vi "tui_LuaVIEW Function Manager.vi"() -> ()   [LabVIEW 2012]
doc: "A manager for Lua-callable functions. It supports LuaVIEW function VIs as well as functions with a doc string contained in function library scripts. The documentation of individual functions can be shown. Overview documentation of the listed functions can be exported to HTML. When running under the LabVIEW development environment, function VIs and their documentation can be opened and edited."
uses:
  served/LuaVIEW Loaded Function Infos_srv.ctl
  served/LuaVIEW Get Function Documentation_srv.ctl
  served/LuaVIEW Cleanup Registry_srv.ctl
  typedefs/t_LuaVIEW Function Manager States.ctl
  library/typedefs/t_Library Session Methods.ctl
  clientsrv/typedefs/t_ClientSrv Access Levels.ctl
  typedefs/clusters/LuaVIEW Function Info.ctl
panel:
  out "cleanup registry":T1
  in  "cleanup":bool
  out "llb path cache":path
  out "new selection":T2(ring)
  out "html paths":path[](array[path])
  out "library path cache":path
  out "base path cache":path
  out "source selection":T2(ring)
  in  "function source":u16(ring) items=["select", "loaded on server", "base directory", "VI library", "function library"]
  out "source":string
  in  "function filter":string
  in  "refresh":bool
  out "get func doc":T3
  in  "edit":bool
  in  "open":bool
  in  "export":bool
  in  "show":bool
  out "loaded func infos":T4
  in  "function list":i32(listbox)
  in  "exit":bool
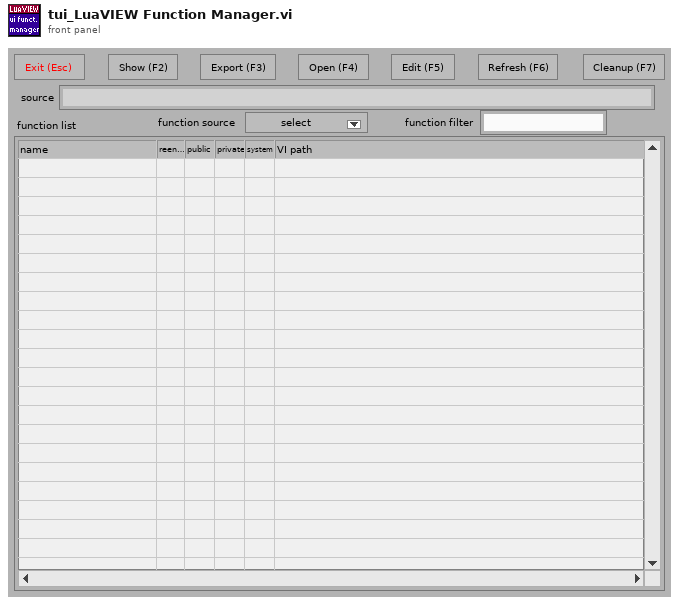
[diagram p1: front panel]
types:
  T1 = typedef "LuaVIEW Cleanup Registry_srv.ctl" = refnum<vi>
  T2 = enum16{"loaded on server", "base directory", "VI library", "function library"}
  T3 = typedef "LuaVIEW Get Function Documentation_srv.ctl" = refnum<vi>
  T4 = typedef "LuaVIEW Loaded Function Infos_srv.ctl" = refnum<vi>
  T5 = typedef "t_LuaVIEW Function Manager States.ctl" = enum16{"empty queue", "update source", "set source", "refresh source", "cleanup registry", "update list", "update ablement", "show", "export", "open", "edit", "fetch loaded", "query base", "query llb", "recurse base", "query library", "parse library", "match sizes", "initialize", "init refs", "init disable", "init persist", "init source", "cleanup", "stop"}
  T6 = typedef "t_Library Session Methods.ctl" = enum16{"run", "get arg", "set arg", "delist", "cleanup?", "start session", "stop session", "list empty?"}
  T7 = typedef "t_ClientSrv Access Levels.ctl" = enum16{"observer", "operator", "local"}
  T8 = typedef "LuaVIEW Function Info.ctl" = cluster{"path":path, "reentrant":bool, "public":bool, "private":i32, "system":bool, "other path":bool, "name":string, "docstring":string, "synopsis":string}
  T9 = typedef "eventvkey.ctl" = enum16{"ASCII", "Enter", "Return", "Shift", "Ctrl", "Alt", "Cmd", "Opt", "Caps", "NumLock", "Clear", "Break", "Up", "Down", "Left", "Right", "Insert", "Delete", "Home", "End", "PageUp", "PageDown", "Escape", "Help", "Pause", "ScrollLock", "F1", "F2", "F3", "F4", "F5", "F6", "F7", "F8", "F9", "F10", "F11", "F12", "F13", "F14", "F15", "F16", "F17", "F18", "F19", "F20", "F21", "F22", "F23", "F24", "Play", "VolumeUp", "VolumeDown", "Mute", "Two Byte Char"}
  T10 = enum32{"invalid app kind", "Development System", "Run Time System", "Student Edition", "Embedded LabVIEW", "Evaluation", "Custom"}
  T11 = enum32{"existing file", "new file", "new or existing file", "existing dir", "new dir", "new or existing dir", "existing file (use LLBs)", "new file (use LLBs)", "new or existing file (use LLBs)", "new or existing file or directory (use LLBs)"}
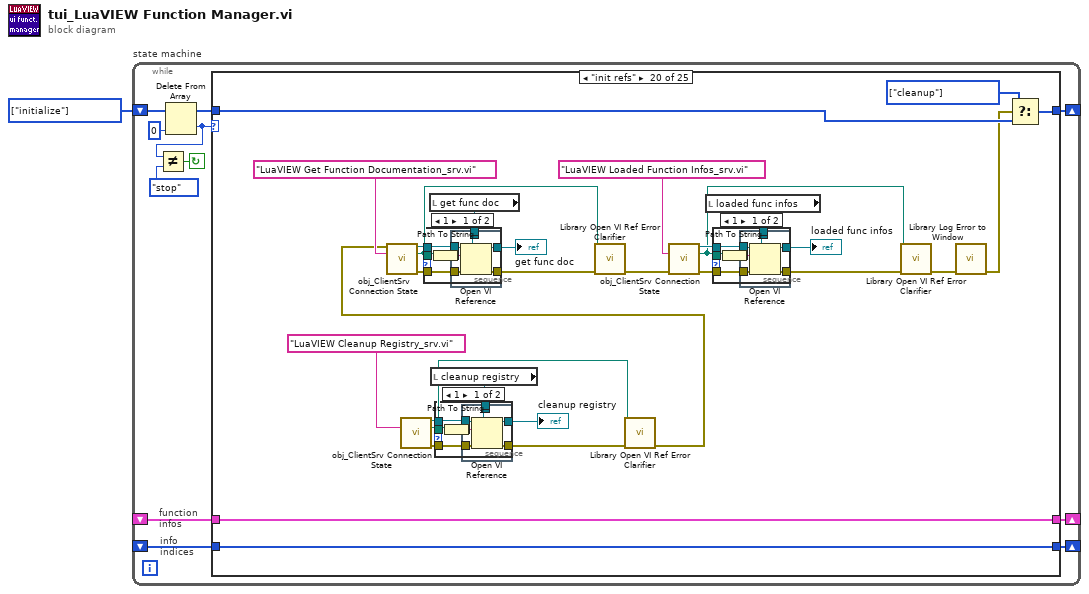
[diagram p0: block diagram]
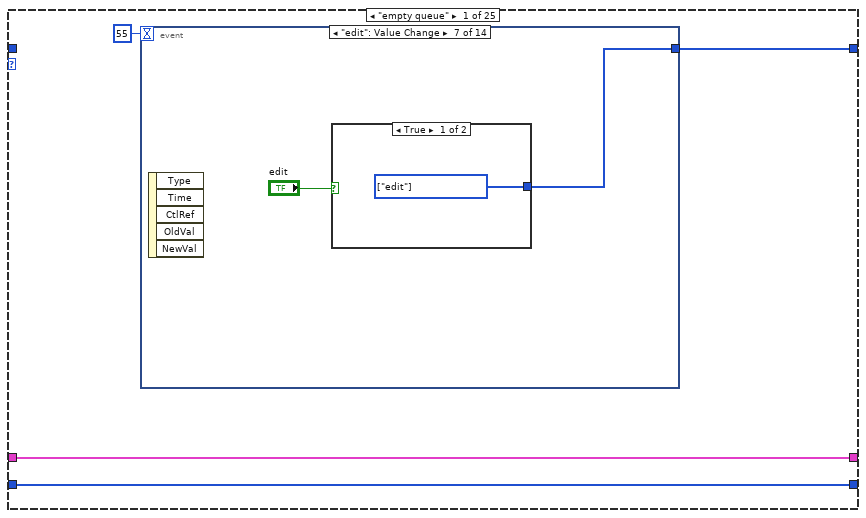
[diagram p2: hidden frame]
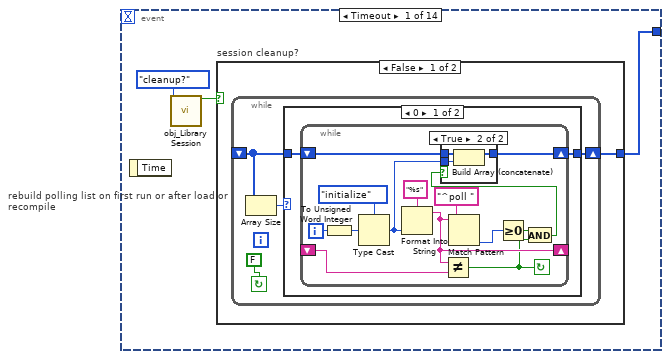
[diagram p3: hidden frame]
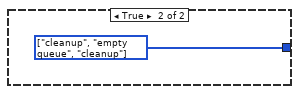
[diagram p6: hidden frame]
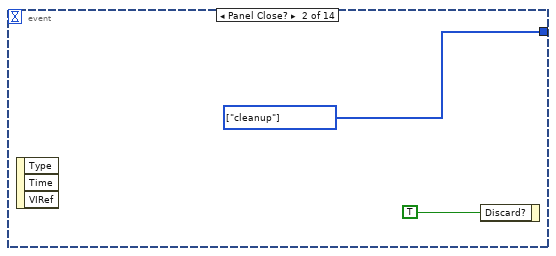
[diagram p7: hidden frame]
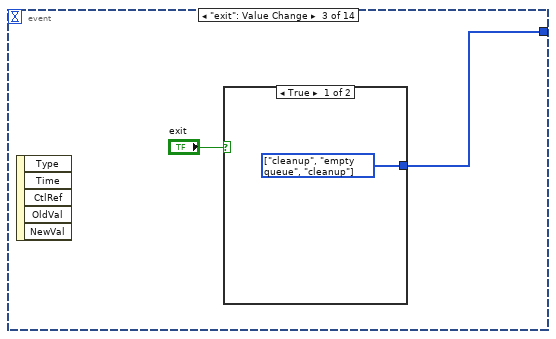
[diagram p8: hidden frame]
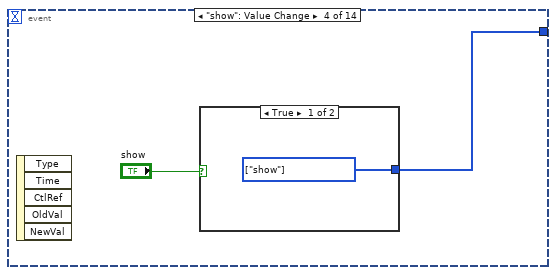
[diagram p10: hidden frame]
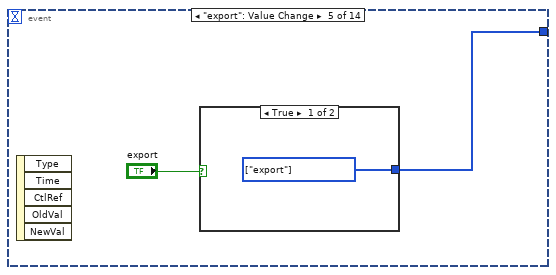
[diagram p12: hidden frame]
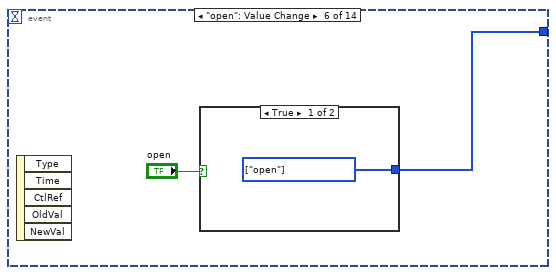
[diagram p14: hidden frame]
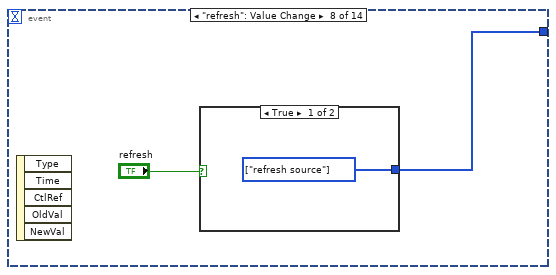
[diagram p17: hidden frame]
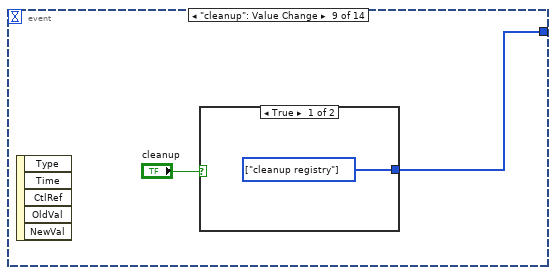
[diagram p19: hidden frame]
diagram:
  w1 = T5[] [enum."initialize"] items=["empty queue", "update source", "set source", "refresh source", "cleanup registry", "update list", "update ablement", "show", "export", "open", "edit", "fetch loaded", "query base", "query llb", "recurse base", "query library", "parse library", "match sizes", "initialize", "init refs", "init disable", "init persist", "init source", "cleanup", "stop"] ("Array Constant")
  n1 = while "state machine" {
    shift-left: w1 -> [w9]
    shift-right: [w12] -> _
    shift-right: [w4] -> _
    shift-left: _ -> [w5]
    shift-right: [w2] -> _
    shift-left: _ -> [w3]
    stop <- w11 continue-if-true
    # "info\nindices"
    # "function\ninfos"
    n2 = Delete From Array(array=w9, index=0) -> (deleted portion=w6:T5, array with subset deleted=w8:T5[])  [unwired: 1 in]
    n3 = Not Equal?(x=w6, y=t_LuaVIEW_Function_Manager_States."stop" ("states")) -> (x != y?=w11:bool)
    n4 = case "Case" shown="\"init refs\"" w6 {
      tunnel: [w16 w98 w105 w109 w124 w141 w214 w231 w268 w380 w394 w405 w430 w443 w453 w477 w488 w502 w507 w562 w629 w631 w651 w660 w663] -> w12
      tunnel: w8 -> [_ _ w105 w108 _ w146 w214 w231 w268 w380 w394 w406 w432 w445 w452 w479 w487 w502 _ w560 w629 w634 w650 _ w663]
      tunnel: w5 -> [w15 w99 w106 w113 w126 w145 w210 w227 w263 w375 w389 _ w431 w444 _ w478 _ w504 w506 w559 w627 w633 w649 w656 w662]
      tunnel: [w15 w99 w106 w113 w126 w145 w210 w227 w263 w375 w389 w407 w431 w444 w454 w478 w489 w504 w506 w559 w627 w633 w647 w656 w662] -> w4
      tunnel: w3 -> [w14 w97 w107 w111 w125 _ w213 w229 w262 w374 w390 w403 w428 w441 w449 w475 w484 w503 w505 w558 w626 w632 w644 w655 w661]
      tunnel: [w14 w97 w107 w111 w125 w142 w213 w229 w262 w374 w390 w403 w428 w441 w449 w475 w484 w503 w505 w558 w626 w632 w643 w655 w661] -> w2
      frame "empty queue" {
        n5 = event shown="[6] \"edit\": Value Change" {
          selector: _ -> [_ _ _ _ _ _ _ _ _ _ _ _ _ _]
          dyn-events: _ -> [_ _ _ _ _ _ _ _ _ _ _ _ _ _]
          timeout: 55 -> [_ _ _ _ _ _ _ _ _ _ _ _ _ _]
          tunnel: [w19 w48 w50 w53 w56 w59 w62 w65 w68 w72 w83 w86 w91 _] -> w16
          event Timeout {
            n6 = event-data() -> ()  [unwired: 1 in, 1 out]
            n7 = call "obj_Library Session.vi"("method"=t_Library_Session_Methods."cleanup?") -> ("cleanup/empty?"=w18:bool)  [unwired: 11 in, 3 out]
            n8 = case "session cleanup?" shown="False" w18 {
              tunnel: [w20 w46] -> w19
              frame False {
                n9 = while "rebuild polling list on first run or after load or recompile" {
                  shift-left: _ -> [w23]
                  shift-right: [w22] -> w20
                  stop <- FALSE continue-if-true
                  n10 = Array Size(array=w23) -> (size(s)=w24:i32)
                  n11 = case shown="0" w24 {
                    tunnel: [w25 w45] -> w22
                    tunnel: w23 -> [w26 w45]
                    frame 0 {
                      n12 = while {
                        shift-left: w26 -> [w35]
                        shift-right: [w33] -> w25
                        shift-left: _ -> [w37]
                        shift-right: [w32] -> _
                        i -> [w40]
                        stop <- w28 continue-if-true
                        n13 = To Unsigned Word Integer(number=w40) -> (unsigned 16bit integer=w38:u16)
                        n14 = Type Cast(type=t_LuaVIEW_Function_Manager_States."initialize" ("states"), x=w38) -> (*(type *) &x=w34:T5)
                        n15 = Format Into String(format string="%s" ("Format String"), w34) -> (resulting string=w32:string)  [unwired: 2 in, 1 out]
                        n16 = Not Equal?(x=w32, y=w37) -> (x != y?=w28:bool)
                        n17 = Match Pattern(string=w32, regular expression="^poll ") -> (offset past match=w30:i32)  [unwired: 1 in, 3 out]
                        n18 = Greater Or Equal To 0?(x=w30) -> (x >= 0?=w29:bool)
                        n19 = And(x=w29, y=w28) -> (x .and. y?=w27:bool)
                        n20 = case shown="True" w27 {
                          tunnel: w35 -> [w41 w44]
                          tunnel: w34 -> [_ w43]
                          tunnel: [w41 w42] -> w33
                          frame False {
                          }
                          frame True {
                            n21 = Build Array (concatenate)(w44, w43) -> (w42:T5[])
                          }
                        }
                      }
                    }
                    frame Default {
                    }
                  }
                }
              }
              frame True {
                w46 = T5[] [enum."cleanup", enum."empty queue", enum."cleanup"] items=["empty queue", "update source", "set source", "refresh source", "cleanup registry", "update list", "update ablement", "show", "export", "open", "edit", "fetch loaded", "query base", "query llb", "recurse base", "query library", "parse library", "match sizes", "initialize", "init refs", "init disable", "init persist", "init source", "cleanup", "stop"] ("Array Constant")
              }
            }
          }
          event Panel Close? {
            w48 = T5[] [enum."cleanup"] items=["empty queue", "update source", "set source", "refresh source", "cleanup registry", "update list", "update ablement", "show", "export", "open", "edit", "fetch loaded", "query base", "query llb", "recurse base", "query library", "parse library", "match sizes", "initialize", "init refs", "init disable", "init persist", "init source", "cleanup", "stop"] ("Array Constant")
            n22 = event-data() -> ()  [unwired: 1 in, 3 out]
            n23 = event-data("Discard?"=TRUE) -> ()  [unwired: 1 in, 1 out]
          }
          event "exit": Value Change {
            n24 = event-data() -> ()  [unwired: 1 in, 5 out]
            n25 = case shown="True" "exit" {
              tunnel: [w51 _] -> w50
              frame True {
                w51 = T5[] [enum."cleanup", enum."empty queue", enum."cleanup"] items=["empty queue", "update source", "set source", "refresh source", "cleanup registry", "update list", "update ablement", "show", "export", "open", "edit", "fetch loaded", "query base", "query llb", "recurse base", "query library", "parse library", "match sizes", "initialize", "init refs", "init disable", "init persist", "init source", "cleanup", "stop"] ("Array Constant")
              }
              frame False {
              }
            }
          }
          event "show": Value Change {
            n26 = event-data() -> ()  [unwired: 1 in, 5 out]
            n27 = case shown="True" "show" {
              tunnel: [w54 _] -> w53
              frame True {
                w54 = T5[] [enum."show"] items=["empty queue", "update source", "set source", "refresh source", "cleanup registry", "update list", "update ablement", "show", "export", "open", "edit", "fetch loaded", "query base", "query llb", "recurse base", "query library", "parse library", "match sizes", "initialize", "init refs", "init disable", "init persist", "init source", "cleanup", "stop"] ("Array Constant")
              }
              frame False {
              }
            }
          }
          event "export": Value Change {
            n28 = event-data() -> ()  [unwired: 1 in, 5 out]
            n29 = case shown="True" "export" {
              tunnel: [w57 _] -> w56
              frame True {
                w57 = T5[] [enum."export"] items=["empty queue", "update source", "set source", "refresh source", "cleanup registry", "update list", "update ablement", "show", "export", "open", "edit", "fetch loaded", "query base", "query llb", "recurse base", "query library", "parse library", "match sizes", "initialize", "init refs", "init disable", "init persist", "init source", "cleanup", "stop"] ("Array Constant")
              }
              frame False {
              }
            }
          }
          event "open": Value Change {
            n30 = event-data() -> ()  [unwired: 1 in, 5 out]
            n31 = case shown="True" "open" {
              tunnel: [w60 _] -> w59
              frame True {
                w60 = T5[] [enum."open"] items=["empty queue", "update source", "set source", "refresh source", "cleanup registry", "update list", "update ablement", "show", "export", "open", "edit", "fetch loaded", "query base", "query llb", "recurse base", "query library", "parse library", "match sizes", "initialize", "init refs", "init disable", "init persist", "init source", "cleanup", "stop"] ("Array Constant")
              }
              frame False {
              }
            }
          }
          event "edit": Value Change {
            n32 = event-data() -> ()  [unwired: 1 in, 5 out]
            n33 = case shown="True" "edit" {
              tunnel: [w63 _] -> w62
              frame True {
                w63 = T5[] [enum."edit"] items=["empty queue", "update source", "set source", "refresh source", "cleanup registry", "update list", "update ablement", "show", "export", "open", "edit", "fetch loaded", "query base", "query llb", "recurse base", "query library", "parse library", "match sizes", "initialize", "init refs", "init disable", "init persist", "init source", "cleanup", "stop"] ("Array Constant")
              }
              frame False {
              }
            }
          }
          event "refresh": Value Change {
            n34 = event-data() -> ()  [unwired: 1 in, 5 out]
            n35 = case shown="True" "refresh" {
              tunnel: [w66 _] -> w65
              frame True {
                w66 = T5[] [enum."refresh source"] items=["empty queue", "update source", "set source", "refresh source", "cleanup registry", "update list", "update ablement", "show", "export", "open", "edit", "fetch loaded", "query base", "query llb", "recurse base", "query library", "parse library", "match sizes", "initialize", "init refs", "init disable", "init persist", "init source", "cleanup", "stop"] ("Array Constant")
              }
              frame False {
              }
            }
          }
          event "cleanup": Value Change {
            n36 = event-data() -> ()  [unwired: 1 in, 5 out]
            n37 = case shown="True" "cleanup" {
              tunnel: [w69 _] -> w68
              frame True {
                w69 = T5[] [enum."cleanup registry"] items=["empty queue", "update source", "set source", "refresh source", "cleanup registry", "update list", "update ablement", "show", "export", "open", "edit", "fetch loaded", "query base", "query llb", "recurse base", "query library", "parse library", "match sizes", "initialize", "init refs", "init disable", "init persist", "init source", "cleanup", "stop"] ("Array Constant")
              }
              frame False {
              }
            }
          }
          event Key Down? {
            n38 = event-data() -> ("VKey"=w70:T9, "FocusObj"=w71:refnum<vi>)  [unwired: 1 in, 6 out]
            n39 = call <vilib>:"compatReturnToEnter.vi"("VKey"=w70) -> ("VKey"=w74:T9)
            n40 = case shown="\"Up\", \"Down\"" w74 {
              tunnel: [_ TRUE TRUE _] -> w73
              tunnel: [_ _ w81 _] -> w72
              tunnel: w71 -> [w76 _ _ _]
              frame "Up", "Down" {
                n41 = Type Cast(type=u32 0, x=w76) -> (*(type *) &x=w77:u32)
                n42 = Equal To 0?(x=w77) -> (x = 0?=w75:bool)
                n43 = case shown="True" w75 {
                  frame False {
                  }
                  frame True {
                    n44 = property on="function list" class="MCListbox (strict)"("Key Focus"=TRUE) -> ()  [unwired: 2 in, 2 out]
                  }
                }
              }
              frame "F1" {
                n45 = call "Library Show Help.vi"() -> ()  [unwired: 1 in]
              }
              frame "Enter" {
                w81 = T5[] [enum."show"] items=["empty queue", "update source", "set source", "refresh source", "cleanup registry", "update list", "update ablement", "show", "export", "open", "edit", "fetch loaded", "query base", "query llb", "recurse base", "query library", "parse library", "match sizes", "initialize", "init refs", "init disable", "init persist", "init source", "cleanup", "stop"] ("Array Constant")
              }
              frame Default {
              }
            }
            n46 = event-data("Discard?"=w73) -> ()  [unwired: 5 in, 1 out]
          }
          event "function filter": Value Change {
            w83 = T5[] [enum."update list"] items=["empty queue", "update source", "set source", "refresh source", "cleanup registry", "update list", "update ablement", "show", "export", "open", "edit", "fetch loaded", "query base", "query llb", "recurse base", "query library", "parse library", "match sizes", "initialize", "init refs", "init disable", "init persist", "init source", "cleanup", "stop"] ("Array Constant")
            n47 = event-data() -> ()  [unwired: 1 in, 5 out]
          }
          event "function source": Value Change {
            n48 = event-data() -> ()  [unwired: 1 in, 6 out]
            n49 = Greater Than 0?(x="function source") -> (x > 0?=w85:bool)
            n50 = case shown="True" w85 {
              tunnel: [_ w89] -> w86
              tunnel: "function source" -> [_ w88]
              frame False {
              }
              frame True {
                w89 = T5[] [enum."update source"] items=["empty queue", "update source", "set source", "refresh source", "cleanup registry", "update list", "update ablement", "show", "export", "open", "edit", "fetch loaded", "query base", "query llb", "recurse base", "query library", "parse library", "match sizes", "initialize", "init refs", "init disable", "init persist", "init source", "cleanup", "stop"] ("Array Constant")
                n51 = Decrement(x=w88) -> (x-1=→"new selection":u16)
                n52 = stacked-sequence {
                  tunnel: w88 -> [_]
                  frame #0 {
                    w90 = u16 0 items=["select", "loaded on server", "base directory", "function library"] ("function source")
                    n53 = local write "function source"(w90) -> ()
                  }
                }
              }
            }
          }
          event Panel Resize {
            w91 = T5[] [enum."match sizes"] items=["empty queue", "update source", "set source", "refresh source", "cleanup registry", "update list", "update ablement", "show", "export", "open", "edit", "fetch loaded", "query base", "query llb", "recurse base", "query library", "parse library", "match sizes", "initialize", "init refs", "init disable", "init persist", "init source", "cleanup", "stop"] ("Array Constant")
            n54 = event-data() -> ()  [unwired: 1 in, 8 out]
          }
          event event type 5.0.x8000000b {
            n55 = event-data() -> ("VKey"=w92:T9)  [unwired: 1 in, 9 out]
            n56 = call <vilib>:"compatReturnToEnter.vi"("VKey"=w92) -> ("VKey"=w94:T9)
            n57 = case shown="\"F1\"" w94 {
              tunnel: [_ TRUE] -> w93
              frame Default {
              }
              frame "F1" {
              }
            }
            n58 = event-data("Discard?"=w93) -> ()  [unwired: 6 in, 1 out]
          }
        }
      }
      frame "update source" {
        n59 = local read "new selection"() -> (w96:T2)
        n60 = case shown="\"VI library\"" w96 {
          tunnel: [w100 w101 w102 w103] -> w98
          frame "loaded on server" {
            w100 = T5[] [enum."set source", enum."fetch loaded"] items=["empty queue", "update source", "set source", "refresh source", "cleanup registry", "update list", "update ablement", "show", "export", "open", "edit", "fetch loaded", "query base", "query llb", "recurse base", "query library", "parse library", "match sizes", "initialize", "init refs", "init disable", "init persist", "init source", "cleanup", "stop"] ("Array Constant")
          }
          frame "base directory" {
            w101 = T5[] [enum."query base"] items=["empty queue", "update source", "set source", "refresh source", "cleanup registry", "update list", "update ablement", "show", "export", "open", "edit", "fetch loaded", "query base", "query llb", "recurse base", "query library", "parse library", "match sizes", "initialize", "init refs", "init disable", "init persist", "init source", "cleanup", "stop"] ("Array Constant")
          }
          frame "VI library" {
            w102 = T5[] [enum."query llb"] items=["empty queue", "update source", "set source", "refresh source", "cleanup registry", "update list", "update ablement", "show", "export", "open", "edit", "fetch loaded", "query base", "query llb", "recurse base", "query library", "parse library", "match sizes", "initialize", "init refs", "init disable", "init persist", "init source", "cleanup", "stop"] ("Array Constant")
          }
          frame "function library" {
            w103 = T5[] [enum."query library"] items=["empty queue", "update source", "set source", "refresh source", "cleanup registry", "update list", "update ablement", "show", "export", "open", "edit", "fetch loaded", "query base", "query llb", "recurse base", "query library", "parse library", "match sizes", "initialize", "init refs", "init disable", "init persist", "init source", "cleanup", "stop"] ("Array Constant")
          }
        }
      }
      frame "set source" {
        n61 = local read "new selection"() -> (→"source selection":T2)
      }
      frame "refresh source" {
        n62 = local read "source selection"() -> (w110:T2)
        n63 = case shown="\"base directory\", \"VI library\"" w110 {
          tunnel: [w114 w115 w116] -> w112
          frame "loaded on server" {
            w114 = T5[] [enum."fetch loaded"] items=["empty queue", "update source", "set source", "refresh source", "cleanup registry", "update list", "update ablement", "show", "export", "open", "edit", "fetch loaded", "query base", "query llb", "recurse base", "query library", "parse library", "match sizes", "initialize", "init refs", "init disable", "init persist", "init source", "cleanup", "stop"] ("Array Constant")
          }
          frame "base directory", "VI library" {
            w115 = T5[] [enum."recurse base"] items=["empty queue", "update source", "set source", "refresh source", "cleanup registry", "update list", "update ablement", "show", "export", "open", "edit", "fetch loaded", "query base", "query llb", "recurse base", "query library", "parse library", "match sizes", "initialize", "init refs", "init disable", "init persist", "init source", "cleanup", "stop"] ("Array Constant")
          }
          frame "function library" {
            w116 = T5[] [enum."parse library"] items=["empty queue", "update source", "set source", "refresh source", "cleanup registry", "update list", "update ablement", "show", "export", "open", "edit", "fetch loaded", "query base", "query llb", "recurse base", "query library", "parse library", "match sizes", "initialize", "init refs", "init disable", "init persist", "init source", "cleanup", "stop"] ("Array Constant")
          }
        }
        n64 = Build Array (concatenate)(w112, w108) -> (w109:T5[])
      }
      frame "cleanup registry" {
        n65 = local read "cleanup registry"() -> (w119:T1)
        n66 = call "obj_ClientSrv Client Access State.vi"("access level (observer)"=t_ClientSrv_Access_Levels."operator") -> ("certificate"=w121:string, "error out"=w120:errorcluster)  [unwired: 13 in]
        n67 = call-by-ref "?"(reference=w119, error in=w120, "certificate"=w121) -> (error out=w122:errorcluster, 15:"error out"=w123:errorcluster)  [unwired: 14 in, 1 out]
        n68 = call "Library Remote Call Error Merger.vi"("call by reference node error"=w122, "called VI error (no error)"=w123) -> ("error out"=w118:errorcluster)  [unwired: 13 in]
        n69 = case shown="No Error" w118 {
          selector: w118 -> [_ w130]
          tunnel: [w127 _] -> w124
          frame No Error {
            n70 = local read "source selection"() -> (w128:T2)
            n71 = case shown="\"loaded on server\"" w128 {
              tunnel: [w129 _] -> w127
              frame "loaded on server" {
                w129 = T5[] [enum."refresh source"] items=["empty queue", "update source", "set source", "refresh source", "cleanup registry", "update list", "update ablement", "show", "export", "open", "edit", "fetch loaded", "query base", "query llb", "recurse base", "query library", "parse library", "match sizes", "initialize", "init refs", "init disable", "init persist", "init source", "cleanup", "stop"] ("Array Constant")
              }
              frame Default {
              }
            }
          }
          frame Error {
            n72 = call "Library Log Error to Window.vi"("error in (no error)"=w130) -> ()  [unwired: 13 in, 2 out]
          }
        }
      }
      frame "update list" {
        # "avoid LV7 bug"
        # "Ignore case and put the non-table functions\nup-front when sorting"
        n73 = Concatenate Strings("function filter", "*" ("string")) -> (w131:string)
        n74 = call "Library Wildcards to Regular.vi"("wildcards"=w131) -> ("regular expression"=w144:string)  [unwired: 4 in]
        n75 = for {
          tunnel: w145 -> [w184] mode=indexing
          tunnel: w144 -> [w198]
          shift-right: [w194] -> w136
          shift-left: cluster{string, "function info":T8, i32}[] [] -> [w181]
          i -> [w182]
          n76 = Unbundle By Name(w184) -> ("name"=w185:string)
          n77 = To Upper Case(1:w185) -> (0:w183:string)
          n78 = Match Pattern(string=w185, regular expression="\\.") -> (offset past match=w191:i32)  [unwired: 1 in, 3 out]
          n79 = Greater Or Equal To 0?(x=w191) -> (x >= 0?=w190:bool)
          n80 = To Upper Case(1:w198) -> (0:w193:string)
          n81 = Select(t="ÿ" ("regular expression"), s=w190, f="") -> (s? t:f=w187:string)
          n82 = Concatenate Strings(w187, w183) -> (w186:string)
          n83 = Match Pattern(string=w183, regular expression=w193) -> (offset past match=w197:i32)  [unwired: 1 in, 3 out]
          n84 = Greater Or Equal To 0?(x=w197) -> (x >= 0?=w196:bool)
          n85 = Bundle(w186, w184, w182) -> (w195:cluster{string, T8, i32})  [unwired: 1 in]
          n86 = case shown="True" w196 {
            tunnel: w181 -> [w199 w202]
            tunnel: w195 -> [_ w201]
            tunnel: [w199 w200] -> w194
            frame False {
            }
            frame True {
              n87 = Build Array (concatenate)(w202, w201) -> (w200:cluster{string, T8, i32}[])
            }
          }
        }
        n88 = local read "source selection"() -> (w138:T2)
        n89 = case shown="\"base directory\", \"VI library\"" w138 {
          tunnel: [_ w148] -> w137
          frame Default {
          }
          frame "base directory", "VI library" {
            n90 = local read "source"() -> (w150:string)
            n91 = String Length(string=w150) -> (length=w149:i32)
            n92 = Increment(x=w149) -> (x+1=w148:i32)
          }
        }
        n93 = Sort 1D Array(array=w136) -> (sorted array=w135:cluster{string, "function info":T8, i32}[])
        n94 = Sort 1D Array(array=w135) -> (sorted array=w134:cluster{string, "function info":T8, i32}[])
        n95 = for {
          tunnel: w134 -> [w180] mode=indexing
          tunnel: [w179] -> w147 mode=indexing
          tunnel: [w174] -> w142 mode=indexing
          tunnel: w137 -> [w172]
          w166 = ""
          n96 = Unbundle(w180) -> ("function info"=w178:T8, w174:i32)  [unwired: 1 out]
          n97 = Unbundle By Name(w178) -> ("name"=w175:string, "reentrant"=w176:bool, "public"=w177:bool, "private"=w173:i32, "system"=w156:bool, "other path"=w155:bool, "path"=w151:path)
          n98 = Strip Path(path=w151) -> (stripped path=w157:path, name=w159:string)
          n99 = Path To String(path=w151) -> (string=w164:string)
          n100 = Format Into String(format string="VI \"%s\" is already loaded from \"%s\"", w159, w157) -> (resulting string=w154:string)  [unwired: 2 in, 1 out]
          n101 = Equal To 0?(x=w173) -> (x = 0?=w167:bool)
          n102 = String Subset(string=w164, offset (0)=w172) -> (substring=w153:string)  [unwired: 1 in]
          n103 = Format Into String(w173) -> (resulting string=w165:string)  [unwired: 3 in, 1 out]
          n104 = Select(t="R", s=w176, f=w166) -> (s? t:f=w168:string)
          n105 = Select(t="P", s=w177, f=w166) -> (s? t:f=w170:string)
          n106 = Select(t=w166, s=w167, f=w165) -> (s? t:f=w171:string)
          n107 = Select(t=w154, s=w155, f=w153) -> (s? t:f=w152:string)
          n108 = Select(t="S", s=w156, f="") -> (s? t:f=w160:string)
          n109 = Build Array(w175, w168, w170, w171, w160, w152) -> (w179:string[])
        }
        n110 = Build Array (concatenate)(t_LuaVIEW_Function_Manager_States."update ablement" ("states"), w146) -> (w141:T5[])
        n111 = property on="function list" class="MCListbox (strict)"("Top Left Visible Cell"=cluster{u32, u32} {0, 0}, "Item Names"=w147) -> ()  [unwired: 2 in, 2 out]
      }
      frame "update ablement" {
        w208 = u8 0 items=["enabled", "disabled", "grayed"] ("disabled state")
        w207 = u8 2 items=["enabled", "disabled", "grayed"] ("disabled state")
        n112 = Array Size(array=w210) -> (size(s)=w211:i32)
        n113 = Greater Than 0?(x=w211) -> (x > 0?=w209:bool)
        n114 = Select(t=w208, s=w209, f=w207) -> (s? t:f=w203:u8)
        n115 = property class="App"() -> ("Application:Kind"=w212:T10)  [unwired: 2 in, 2 out]
        n116 = property on="export" class="Bool"("Disabled"=w203) -> ()  [unwired: 2 in, 2 out]
        n117 = property on="show" class="Bool"("Disabled"=w203) -> ()  [unwired: 2 in, 2 out]
        n118 = case shown="\"Run Time System\"" w212 {
          tunnel: w203 -> [w217 _]
          tunnel: w207 -> [_ w218]
          tunnel: [w217 w218] -> w205
          frame Default {
          }
          frame "Run Time System" {
          }
        }
        n119 = local read "source selection"() -> (w206:T2)
        n120 = case shown="Default" w206 {
          tunnel: w207 -> [w215 _]
          tunnel: w205 -> [_ w216]
          tunnel: [w215 w216] -> w204
          frame "function library" {
          }
          frame Default {
          }
        }
        n121 = property on="open" class="Bool"("Disabled"=w204) -> ()  [unwired: 2 in, 2 out]
        n122 = property on="edit" class="Bool"("Disabled"=w204) -> ()  [unwired: 2 in, 2 out]
      }
      frame "show" {
        n123 = Index Array(array=w229, index="function list") -> (element=w228:i32)
        n124 = local read "source selection"() -> (w222:T2)
        n125 = Index Array(array=w227, index=w228) -> (element=w226:T8)
        n126 = case shown="\"base directory\", \"VI library\"" w222 {
          tunnel: w226 -> [w237 w239 w251]
          tunnel: [_ w242 w253] -> w221
          tunnel: [w237 w241 w252] -> w220
          frame "function library" {
          }
          frame "loaded on server" {
            n127 = Unbundle By Name(w239) -> ("path"=w238:path)
            n128 = call "obj_ClientSrv Client Access State.vi"() -> ("certificate"=w247:string, "error out"=w246:errorcluster)  [unwired: 14 in]
            n129 = local read "get func doc"() -> (w240:T3)
            n130 = call-by-ref "?"(reference=w240, error in=w246, "function path"=w238, "certificate"=w247) -> (error out=w248:errorcluster, "documentation"=w245:string, "reentrant?"=w244:bool, "synopsis"=w243:string, 15:"error out"=w249:errorcluster)  [unwired: 10 in, 1 out]
            n131 = call "Library Remote Call Error Merger.vi"("call by reference node error"=w248, "called VI error (no error)"=w249) -> ("error out"=w242:errorcluster)  [unwired: 13 in]
            n132 = Bundle By Name(cluster=w239, "docstring"=w245, "reentrant"=w244, "synopsis"=w243) -> (w241:T8)
          }
          frame "base directory", "VI library" {
            n133 = Unbundle By Name(w251) -> ("path"=w250:path)
            n134 = call "LuaVIEW Get Function Documentation.vi"("function path"=w250) -> ("documentation"=w256:string, "reentrant?"=w255:bool, "synopsis"=w254:string, "error out"=w253:errorcluster)  [unwired: 11 in]
            n135 = Bundle By Name(cluster=w251, "docstring"=w256, "reentrant"=w255, "synopsis"=w254) -> (w252:T8)
          }
        }
        n136 = Flatten To String(anything=w220) -> (data string=w219:string)  [unwired: 3 in, 2 out]
        n137 = call "Library Resolve VI Path.vi"("VI name"="ui_LuaVIEW Show Function Documentation.vit", "sub path of toolkit (none)"=path "dynamic" ("subdirectory of tree (none)")) -> ("VI path"=w225:path)  [unwired: 13 in]
        n138 = case shown="No Error" w221 {
          selector: w221 -> [_ w236]
          tunnel: w225 -> [w234 _]
          tunnel: w219 -> [w232 _]
          frame No Error {
            n139 = call "obj_Library Session.vi"("method"=t_Library_Session_Methods."run", "path"=w234, "argument in (none)"=w232) -> ("error out"=w233:errorcluster)  [unwired: 9 in, 3 out]
            n140 = call "Library Log Error to Window.vi"("error in (no error)"=w233) -> ()  [unwired: 13 in, 2 out]
          }
          frame Error {
            n141 = call "Library Log Error to Window.vi"("error in (no error)"=w236) -> ()  [unwired: 13 in, 2 out]
          }
        }
      }
      frame "export" {
        n142 = local read "source selection"() -> (w260:T2)
        n143 = case shown="\"base directory\", \"VI library\"" w260 {
          tunnel: [w276 w304 w332] -> w267
          tunnel: [w275 w303 w331] -> w266
          tunnel: [w274 w310 w336] -> w265
          tunnel: [w273 w309 w335] -> w264
          tunnel: w263 -> [w272 w308 w334]
          tunnel: w262 -> [w271 w307 w333]
          tunnel: [w269 w305 FALSE ("error?")] -> w261
          frame "loaded on server" {
            n144 = call "obj_ClientSrv Client Access State.vi"() -> ("certificate"=w278:string, "error out"=w277:errorcluster)  [unwired: 14 in]
            n145 = stacked-sequence {
              tunnel: w278 -> [_ w287 _]
              tunnel: w277 -> [_ w286 _]
              tunnel: [_ w285 _] -> w270
              tunnel: [_ w284 _] -> w276
              tunnel: [_ w283 _] -> w275
              tunnel: [_ w282 _] -> w274
              tunnel: [_ w281 _] -> w273
              tunnel: w272 -> [_ w280 _]
              tunnel: w271 -> [_ w279 _]
              frame #0 {
                n146 = call <vilib>:"Set Busy.vi"() -> ()  [unwired: 10 in, 2 out]
              }
              frame #1 {
                n147 = for {
                  tunnel: w287 -> [w300]
                  shift-right: [w299] -> w285
                  shift-left: w286 -> [w298]
                  tunnel: [w297] -> w284 mode=indexing
                  tunnel: [w296] -> w283 mode=indexing
                  tunnel: [w294] -> w282 mode=indexing
                  tunnel: [w289] -> w281 mode=indexing
                  tunnel: w280 -> [w293]
                  tunnel: w279 -> [w292] mode=indexing
                  n148 = local read "get func doc"() -> (w288:T3)
                  n149 = Index Array(array=w293, index=w292) -> (element=w291:T8)
                  n150 = Unbundle By Name(w291) -> ("path"=w290:path, "name"=w289:string)
                  n151 = call-by-ref "?"(reference=w288, error in=w298, "function path"=w290, "certificate"=w300) -> (error out=w301:errorcluster, "documentation"=w297:string, "reentrant?"=w296:bool, "synopsis"=w295:string, 15:"error out"=w302:errorcluster)  [unwired: 10 in, 1 out]
                  n152 = Format Into String(format string=w295, w289) -> (resulting string=w294:string)  [unwired: 2 in, 1 out]
                  n153 = call "Library Remote Call Error Merger.vi"("call by reference node error"=w301, "called VI error (no error)"=w302) -> ("error out"=w299:errorcluster)  [unwired: 13 in]
                }
              }
              frame #2 {
                n154 = call <vilib>:"Unset Busy.vi"() -> ()  [unwired: 11 in, 1 out]
              }
            }
            n155 = call "Library Log Error to Window.vi"("error in (no error)"=w270) -> ("error?"=w269:bool)  [unwired: 13 in, 1 out]
          }
          frame "base directory", "VI library" {
            n156 = stacked-sequence {
              tunnel: [_ w318 _] -> w306
              tunnel: [_ w317 _] -> w303
              tunnel: [_ w316 _] -> w304
              tunnel: [_ w315 _] -> w310
              tunnel: [_ w314 _] -> w309
              tunnel: w308 -> [_ w313 _]
              tunnel: w307 -> [_ w312 _]
              frame #0 {
                n157 = call <vilib>:"Set Busy.vi"() -> ()  [unwired: 10 in, 2 out]
              }
              frame #1 {
                n158 = for {
                  shift-right: [w323] -> w318
                  shift-left: errorcluster {"status"=FALSE, "code"=0, "source"=""} ("error out") -> [w322]
                  tunnel: [w329] -> w317 mode=indexing
                  tunnel: [w325] -> w316 mode=indexing
                  tunnel: [w321] -> w315 mode=indexing
                  tunnel: [w319] -> w314 mode=indexing
                  tunnel: w313 -> [w328]
                  tunnel: w312 -> [w327] mode=indexing
                  n159 = Index Array(array=w328, index=w327) -> (element=w326:T8)
                  n160 = Unbundle By Name(w326) -> ("path"=w324:path, "name"=w319:string)
                  n161 = call "LuaVIEW Get Function Documentation.vi"("function path"=w324, "error in (no error)"=w322) -> ("documentation"=w325:string, "reentrant?"=w329:bool, "synopsis"=w320:string, "error out"=w323:errorcluster)  [unwired: 10 in]
                  n162 = Format Into String(format string=w320, w319) -> (resulting string=w321:string)  [unwired: 2 in, 1 out]
                }
              }
              frame #2 {
                n163 = call <vilib>:"Unset Busy.vi"() -> ()  [unwired: 11 in, 1 out]
              }
            }
            n164 = call "Library Log Error to Window.vi"("error in (no error)"=w306) -> ("error?"=w305:bool)  [unwired: 13 in, 1 out]
          }
          frame "function library" {
            n165 = for {
              tunnel: [FALSE] -> w331 mode=indexing
              tunnel: [w341] -> w332 mode=indexing
              tunnel: [w338] -> w336 mode=indexing
              tunnel: [w337] -> w335 mode=indexing
              tunnel: w334 -> [w344]
              tunnel: w333 -> [w343] mode=indexing
              n166 = Index Array(array=w344, index=w343) -> (element=w342:T8)
              n167 = Unbundle By Name(w342) -> ("docstring"=w341:string, "synopsis"=w339:string, "name"=w337:string)
              n168 = Format Into String(format string=w339, w337) -> (resulting string=w338:string)  [unwired: 2 in, 1 out]
            }
          }
        }
        n169 = local read "html paths"() -> (w259:path[])
        n170 = To Long Integer(number=w260) -> (32bit integer=w257:i32)
        n171 = Index Array(array=w259, index=w257) -> (element=w258:path)
        n172 = case shown="False" w261 {
          tunnel: w267 -> [w357 _]
          tunnel: w266 -> [w355 _]
          tunnel: w265 -> [w354 _]
          tunnel: w264 -> [w353 _]
          tunnel: w258 -> [w347 _]
          tunnel: w257 -> [w346 _]
          frame False {
            (unwired) T11."new or existing file" ("select mode (2)")
            n173 = local read "function filter"() -> (w356:string)
            n174 = local read "source"() -> (w345:string)
            n175 = call "LuaVIEW Format HTML Function List.vi"("filter"=w356, "source"=w345, "names"=w353, "synopses"=w354, "docstrings"=w357, "reentrancy flags"=w355) -> ("HTML list"=w348:string)  [unwired: 9 in]
            n176 = File Dialog(6:"*.html" ("pattern"), 7:"Specify an HTML file to export to" ("prompt (default)"), 11:w347) -> (1:w350:bool, 3:w349:path)  [unwired: 4 in, 2 out]
            n177 = case "cancelled?" shown="False" w350 {
              tunnel: w349 -> [w360 _]
              tunnel: w348 -> [w363 _]
              tunnel: w346 -> [w359 _]
              frame False {
                n178 = call "Library Write Text File.vi"("file path"=w360, "text to write"=w363) -> ("dup path"=w358:path, "error out"=w364:errorcluster)  [unwired: 12 in]
                n179 = local read "html paths"() -> (w362:path[])
                n180 = case shown="No Error" w364 {
                  selector: w364 -> [_ w372]
                  tunnel: w358 -> [w365 _]
                  frame No Error {
                    n181 = Two Button Dialog(message="Do you want to browse the exported documentation?" ("file extension (none required)"), 1:"No" ("file extension (none required)"), 2:"Yes" ("file extension (none required)")) -> (T button?=w369:bool)
                    n182 = case shown="True" w369 {
                      tunnel: w365 -> [_ w370]
                      frame False {
                      }
                      frame True {
                        n183 = call <vilib>:"Open URL in Default Browser (path).vi"("path"=w370) -> ("error out"=w371:errorcluster)  [unwired: 5 in, 1 out]
                        n184 = call "Library Log Error to Window.vi"("error in (no error)"=w371) -> ()  [unwired: 13 in, 2 out]
                      }
                    }
                  }
                  frame Error {
                    n185 = call "Library Log Error to Window.vi"("error in (no error)"=w372) -> ()  [unwired: 13 in, 2 out]
                  }
                }
                n186 = Replace Array Subset(array=w362, new element=w360, index=w359) -> (→"html paths":path[])
              }
              frame True {
              }
            }
          }
          frame True {
          }
        }
      }
      frame "open" {
        n187 = local read "function list"() -> (w373:i32)
        n188 = Index Array(array=w374, index=w373) -> (element=w378:i32)
        n189 = Index Array(array=w375, index=w378) -> (element=w377:T8)
        n190 = Unbundle By Name(w377) -> ("path"=w376:path)
        n191 = Empty String/Path?(string/path=w376) -> (empty?=w379:bool)
        n192 = case shown="False" w379 {
          tunnel: w376 -> [w383 _]
          frame False {
            n193 = Open VI Reference(vi path=w383) -> (vi reference=w386:refnum<vi>, error out=w384:errorcluster)  [unwired: 5 in]
            n194 = call "Library Open VI Ref Error Clarifier.vi"("VI path"=w383, "called VI error (no error)"=w384) -> ("error out"=w382:errorcluster)  [unwired: 13 in]
            n195 = invoke class="VI" method="FP.Old Open"(reference=w386, error in=w382) -> (reference out=w385:refnum<vi>, error out=w381:errorcluster)  [unwired: 3 in, 3 out]
            n196 = Close Reference(reference=w385) -> ()  [unwired: 1 in, 1 out]
            n197 = call "Library Log Error to Window.vi"("error in (no error)"=w381) -> ()  [unwired: 13 in, 2 out]
          }
          frame True {
          }
        }
      }
      frame "edit" {
        n198 = local read "function list"() -> (w388:i32)
        n199 = Index Array(array=w390, index=w388) -> (element=w392:i32)
        n200 = Index Array(array=w389, index=w392) -> (element=w391:T8)
        n201 = Unbundle By Name(w391) -> ("path"=w387:path)
        n202 = Empty String/Path?(string/path=w387) -> (empty?=w393:bool)
        n203 = case shown="False" w393 {
          tunnel: w387 -> [w397 _]
          frame False {
            n204 = Path To String(path=w397) -> (string=w395:string)
            n205 = call "Library Resolve VI Path.vi"("VI name"="ui_LuaVIEW Edit Function Documentation.vit", "sub path of toolkit (none)"=path "dynamic/do not build" ("subdirectory of tree (none)")) -> ("VI path"=w400:path)  [unwired: 13 in]
            n206 = call "obj_Library Session.vi"("method"=t_Library_Session_Methods."run", "path"=w400, "argument in (none)"=w395) -> ("error out"=w398:errorcluster)  [unwired: 9 in, 3 out]
            n207 = call "Library Log Error to Window.vi"("error in (no error)"=w398) -> ()  [unwired: 13 in, 2 out]
          }
          frame True {
          }
        }
      }
      frame "fetch loaded" {
        w402 = T5[] [enum."update list"] items=["empty queue", "update source", "set source", "refresh source", "cleanup registry", "update list", "update ablement", "show", "export", "open", "edit", "fetch loaded", "query base", "query llb", "recurse base", "query library", "parse library", "match sizes", "initialize", "init refs", "init disable", "init persist", "init source", "cleanup", "stop"] ("Array Constant")
        n208 = flat-sequence {
          tunnel: [w411] -> w404
          tunnel: [w423] -> w407
          tunnel: w404 -> [w423]
          frame #0 {
            n209 = call <vilib>:"Set Busy.vi"() -> ()  [unwired: 10 in, 2 out]
          }
          frame #1 {
            n210 = local read "loaded func infos"() -> (w408:T4)
            n211 = call "obj_ClientSrv Client Access State.vi"() -> ("certificate"=w414:string, "error out"=w413:errorcluster)  [unwired: 14 in]
            n212 = call-by-ref "?"(reference=w408, error in=w413, "certificate"=w414) -> (error out=w417:errorcluster, "function infos"=w412:T8[], 15:"error out"=w415:errorcluster)  [unwired: 13 in, 1 out]
            n213 = call "Library Remote Call Error Merger.vi"("call by reference node error"=w417, "called VI error (no error)"=w415) -> ("error out"=w416:errorcluster)  [unwired: 13 in]
            n214 = call "Library Log Error to Window.vi"("error in (no error)"=w416) -> ("error?"=w410:bool)  [unwired: 13 in, 1 out]
            n215 = case shown="False" w410 {
              tunnel: w412 -> [w421 _]
              tunnel: [w421 _] -> w411
              tunnel: [w418 "Error on querying server for loaded function VIs"] -> w409
              frame False {
                n216 = call "obj_ClientSrv Connection State.vi"() -> ("server"=w420:string)  [unwired: 8 in, 7 out]
                n217 = Format Into String(format string="Function VIs loaded on server \"%s\"", w420) -> (resulting string=w418:string)  [unwired: 2 in, 1 out]
              }
              frame True {
              }
            }
            n218 = local write "source"(w409) -> ()
          }
          frame #2 {
            n219 = call <vilib>:"Unset Busy.vi"() -> ()  [unwired: 11 in, 1 out]
          }
        }
        n220 = Build Array (concatenate)(w402, w406) -> (w405:T5[])
      }
      frame "query base" {
        (unwired) T11."existing dir" ("select mode (2)")
        n221 = local read "base path cache"() -> (w425:path)
        n222 = File Dialog(7:"Please select a base directory containing function VIs" ("prompt (default)"), 11:w425) -> (1:w426:bool, 3:w424:path)  [unwired: 5 in, 2 out]
        n223 = case "cancelled?" shown="False" w426 {
          tunnel: w424 -> [w433 _]
          tunnel: [w435 _] -> w429
          frame False {
            w435 = T5[] [enum."set source", enum."recurse base"] items=["empty queue", "update source", "set source", "refresh source", "cleanup registry", "update list", "update ablement", "show", "export", "open", "edit", "fetch loaded", "query base", "query llb", "recurse base", "query library", "parse library", "match sizes", "initialize", "init refs", "init disable", "init persist", "init source", "cleanup", "stop"] ("Array Constant")
            n224 = Path To String(path=w433) -> (string=→"source":string)
            "base path cache" <- w433
          }
          frame True {
          }
        }
        n225 = Build Array (concatenate)(w429, w432) -> (w430:T5[])
      }
      frame "query llb" {
        (unwired) T11."existing file" ("select mode (2)")
        n226 = local read "llb path cache"() -> (w438:path)
        n227 = File Dialog(6:"*.llb" ("pattern"), 7:"Please select an llb containing function VIs" ("prompt (default)"), 11:w438) -> (1:w439:bool, 3:w437:path)  [unwired: 4 in, 2 out]
        n228 = case "cancelled?" shown="False" w439 {
          tunnel: w437 -> [w447 _]
          tunnel: [w448 _] -> w442
          frame False {
            w448 = T5[] [enum."set source", enum."recurse base"] items=["empty queue", "update source", "set source", "refresh source", "cleanup registry", "update list", "update ablement", "show", "export", "open", "edit", "fetch loaded", "query base", "query llb", "recurse base", "query library", "parse library", "match sizes", "initialize", "init refs", "init disable", "init persist", "init source", "cleanup", "stop"] ("Array Constant")
            n229 = Path To String(path=w447) -> (string=w446:string)
            n230 = local write "source"(w446) -> ()
            "llb path cache" <- w447
          }
          frame True {
          }
        }
        n231 = Build Array (concatenate)(w442, w445) -> (w443:T5[])
      }
      frame "recurse base" {
        n232 = flat-sequence {
          tunnel: [w456] -> w450
          tunnel: [w469] -> w454
          tunnel: w450 -> [w469]
          frame #0 {
            n233 = call <vilib>:"Set Busy.vi"() -> ()  [unwired: 10 in, 2 out]
          }
          frame #1 {
            n234 = local read "source"() -> (w462:string)
            n235 = String To Path(string=w462) -> (path=w455:path)
            n236 = call "Library Recursively List Files.vi"("root directory"=w455, "pattern (none)"="*_lua.vi" ("pattern")) -> ("file list"=w461:path[], "error out"=w460:errorcluster)  [unwired: 11 in, 1 out]
            n237 = for {
              tunnel: w461 -> [w468] mode=indexing
              shift-right: [w466] -> w457
              shift-left: w460 -> [w467]
              tunnel: [w465] -> w458 mode=indexing
              n238 = call "LuaVIEW Get Function Info.vi"("function VI path"=w468, "error in (no error)"=w467) -> ("function info"=w465:T8, "error out"=w466:errorcluster)  [unwired: 12 in]
            }
            n239 = call "Library Log Error to Window.vi"("error in (no error)"=w457) -> ("error?"=w459:bool)  [unwired: 13 in, 1 out]
            n240 = case shown="True" w459 {
              tunnel: w458 -> [w464 _]
              tunnel: [w464 _] -> w456
              frame False {
              }
              frame True {
              }
            }
          }
          frame #2 {
            n241 = call <vilib>:"Unset Busy.vi"() -> ()  [unwired: 11 in, 1 out]
          }
        }
        n242 = Build Array (concatenate)(t_LuaVIEW_Function_Manager_States."update list" ("states"), w452) -> (w453:T5[])
      }
      frame "query library" {
        (unwired) T11."existing file" ("select mode (2)")
        n243 = local read "library path cache"() -> (w470:path)
        n244 = File Dialog(6:"*.lua" ("pattern"), 7:"Please select a function library script" ("prompt (default)"), 11:w470) -> (1:w472:bool, 3:w473:path)  [unwired: 4 in, 2 out]
        n245 = case "cancelled?" shown="False" w472 {
          tunnel: w473 -> [w481 _]
          tunnel: [w483 _] -> w476
          frame False {
            w483 = T5[] [enum."set source", enum."parse library"] items=["empty queue", "update source", "set source", "refresh source", "cleanup registry", "update list", "update ablement", "show", "export", "open", "edit", "fetch loaded", "query base", "query llb", "recurse base", "query library", "parse library", "match sizes", "initialize", "init refs", "init disable", "init persist", "init source", "cleanup", "stop"] ("Array Constant")
            n246 = local read "new selection"() -> (w480:T2)
            n247 = Path To String(path=w481) -> (string=w482:string)
            n248 = local write "source"(w482) -> ()
            n249 = local write "source selection"(w480) -> ()
            "library path cache" <- w481
          }
          frame True {
          }
        }
        n250 = Build Array (concatenate)(w476, w479) -> (w477:T5[])
      }
      frame "parse library" {
        n251 = flat-sequence {
          tunnel: [w494] -> w485
          tunnel: [w497] -> w489
          tunnel: w485 -> [w497]
          frame #0 {
            n252 = call <vilib>:"Set Busy.vi"() -> ()  [unwired: 10 in, 2 out]
          }
          frame #1 {
            n253 = local read "source"() -> (w493:string)
            n254 = String To Path(string=w493) -> (path=w492:path)
            n255 = call "LuaVIEW Parse Library Infos.vi"("library path"=w492) -> ("library infos"=w490:T8[], "error out"=w491:errorcluster)  [unwired: 13 in]
            n256 = call "Library Log Error to Window.vi"("error in (no error)"=w491) -> ("error?"=w495:bool)  [unwired: 13 in, 1 out]
            n257 = case shown="False" w495 {
              tunnel: w490 -> [w496 _]
              tunnel: [w496 _] -> w494
              frame False {
              }
              frame True {
              }
            }
          }
          frame #2 {
            n258 = call <vilib>:"Unset Busy.vi"() -> ()  [unwired: 11 in, 1 out]
          }
        }
        n259 = Build Array (concatenate)(t_LuaVIEW_Function_Manager_States."update list" ("states"), w487) -> (w488:T5[])
      }
      frame "match sizes" {
        n260 = property on="function list" class="MCListbox (strict)"() -> ("Position:Left"=w499:i32, "Bounds:Width"=w501:u32)  [unwired: 2 in, 2 out]
        n261 = Subtract(x=w501, y=u32 55) -> (x-y=w498:u32)
        n262 = property on="source" class="Str"("Position:Left"=w499, "Size:Width"=w498) -> ()  [unwired: 2 in, 2 out]
      }
      frame "initialize" {
        n263 = while "rebuild init list on first run or after load or recompile" {
          shift-left: _ -> [w510]
          shift-right: [w509] -> w507
          stop <- FALSE continue-if-true
          n264 = Array Size(array=w510) -> (size(s)=w511:i32)
          n265 = case shown="0" w511 {
            tunnel: [w512 w532] -> w509
            tunnel: w510 -> [w513 w532]
            frame 0 {
              n266 = while {
                shift-left: w513 -> [w522]
                shift-right: [w520] -> w512
                shift-left: _ -> [w524]
                shift-right: [w519] -> _
                i -> [w527]
                stop <- w515 continue-if-true
                n267 = To Unsigned Word Integer(number=w527) -> (unsigned 16bit integer=w525:u16)
                n268 = Type Cast(type=t_LuaVIEW_Function_Manager_States."initialize" ("states"), x=w525) -> (*(type *) &x=w521:T5)
                n269 = Format Into String(format string="%s" ("Format String"), w521) -> (resulting string=w519:string)  [unwired: 2 in, 1 out]
                n270 = Not Equal?(x=w519, y=w524) -> (x != y?=w515:bool)
                n271 = Match Pattern(string=w519, regular expression="^init ") -> (offset past match=w517:i32)  [unwired: 1 in, 3 out]
                n272 = Greater Or Equal To 0?(x=w517) -> (x >= 0?=w516:bool)
                n273 = And(x=w516, y=w515) -> (x .and. y?=w514:bool)
                n274 = case shown="True" w514 {
                  tunnel: w522 -> [w528 w531]
                  tunnel: w521 -> [_ w530]
                  tunnel: [w528 w529] -> w520
                  frame False {
                  }
                  frame True {
                    n275 = Build Array (concatenate)(w531, w530) -> (w529:T5[])
                  }
                }
              }
            }
            frame Default {
            }
          }
        }
      }
      frame "init refs" {
        w561 = T5[] [enum."cleanup"] items=["empty queue", "update source", "set source", "refresh source", "cleanup registry", "update list", "update ablement", "show", "export", "open", "edit", "fetch loaded", "query base", "query llb", "recurse base", "query library", "parse library", "match sizes", "initialize", "init refs", "init disable", "init persist", "init source", "cleanup", "stop"] ("Array Constant")
        n276 = call "obj_ClientSrv Connection State.vi"("machine{connect}/VI{get state} name (local/no path resolution)"="LuaVIEW Cleanup Registry_srv.vi") -> ("server app ref"=w546:refnum<vi>, "resolved server path"=w545:path, "error out"=w547:errorcluster)  [unwired: 7 in, 5 out]
        n277 = local read "get func doc"() -> (w540:T3)
        n278 = local read "cleanup registry"() -> (w549:T1)
        n279 = stacked-sequence {
          tunnel: [w610] -> w548
          tunnel: [w609] -> w550
          tunnel: w547 -> [w608]
          tunnel: w546 -> [w607]
          tunnel: w545 -> [w606]
          tunnel: w549 -> [w605]
          frame #0 {
            # "avoid LV8 complaints"
            n280 = Path to Array of Strings(0:w606) -> (2:w611:string[])  [unwired: 1 out]
            n281 = Array Size(array=w611) -> (size(s)=w612:i32)
            n282 = case shown="1" w612 {
              tunnel: w606 -> [w619 w625]
              tunnel: w607 -> [w617 w624]
              tunnel: [w615 w620] -> w610
              tunnel: [w613 w623] -> w609
              tunnel: w605 -> [w614 w622]
              tunnel: w608 -> [w616 w621]
              frame 1 {
                n283 = Path To String(path=w619) -> (string=w618:string)
                n284 = Open VI Reference(type specifier VI Refnum (for type only)=w614, application reference (local)=w617, vi path=w618, error in (no error)=w616) -> (vi reference=w615:T1, error out=w613:errorcluster)  [unwired: 2 in]
              }
              frame Default {
                n285 = Open VI Reference(type specifier VI Refnum (for type only)=w622, application reference (local)=w624, vi path=w625, error in (no error)=w621) -> (vi reference=w620:T1, error out=w623:errorcluster)  [unwired: 2 in]
              }
            }
          }
        }
        "cleanup registry" <- w548
        n286 = call "Library Open VI Ref Error Clarifier.vi"("VI path"=w545, "called VI error (no error)"=w550) -> ("error out"=w551:errorcluster)  [unwired: 13 in]
        n287 = call "obj_ClientSrv Connection State.vi"("machine{connect}/VI{get state} name (local/no path resolution)"="LuaVIEW Get Function Documentation_srv.vi", "error in (no error)"=w551) -> ("server app ref"=w542:refnum<vi>, "resolved server path"=w541:path, "error out"=w543:errorcluster)  [unwired: 6 in, 5 out]
        n288 = stacked-sequence {
          tunnel: [w589] -> w539
          tunnel: [w588] -> w544
          tunnel: w543 -> [w587]
          tunnel: w542 -> [w586]
          tunnel: w541 -> [w585]
          tunnel: w540 -> [w584]
          frame #0 {
            # "avoid LV8 complaints"
            n289 = Path to Array of Strings(0:w585) -> (2:w590:string[])  [unwired: 1 out]
            n290 = Array Size(array=w590) -> (size(s)=w591:i32)
            n291 = case shown="1" w591 {
              tunnel: w585 -> [w598 w604]
              tunnel: w586 -> [w596 w603]
              tunnel: [w594 w599] -> w589
              tunnel: [w592 w602] -> w588
              tunnel: w584 -> [w593 w601]
              tunnel: w587 -> [w595 w600]
              frame 1 {
                n292 = Path To String(path=w598) -> (string=w597:string)
                n293 = Open VI Reference(type specifier VI Refnum (for type only)=w593, application reference (local)=w596, vi path=w597, error in (no error)=w595) -> (vi reference=w594:T3, error out=w592:errorcluster)  [unwired: 2 in]
              }
              frame Default {
                n294 = Open VI Reference(type specifier VI Refnum (for type only)=w601, application reference (local)=w603, vi path=w604, error in (no error)=w600) -> (vi reference=w599:T3, error out=w602:errorcluster)  [unwired: 2 in]
              }
            }
          }
        }
        "get func doc" <- w539
        n295 = call "Library Open VI Ref Error Clarifier.vi"("VI path"=w541, "called VI error (no error)"=w544) -> ("error out"=w555:errorcluster)  [unwired: 13 in]
        n296 = call "obj_ClientSrv Connection State.vi"("machine{connect}/VI{get state} name (local/no path resolution)"="LuaVIEW Loaded Function Infos_srv.vi", "error in (no error)"=w555) -> ("server app ref"=w536:refnum<vi>, "resolved server path"=w535:path, "error out"=w534:errorcluster)  [unwired: 6 in, 5 out]
        n297 = local read "loaded func infos"() -> (w533:T4)
        n298 = stacked-sequence {
          tunnel: [w568] -> w537
          tunnel: [w567] -> w538
          tunnel: w534 -> [w566]
          tunnel: w536 -> [w565]
          tunnel: w535 -> [w564]
          tunnel: w533 -> [w563]
          frame #0 {
            # "avoid LV8 complaints"
            n299 = Path to Array of Strings(0:w564) -> (2:w569:string[])  [unwired: 1 out]
            n300 = Array Size(array=w569) -> (size(s)=w570:i32)
            n301 = case shown="1" w570 {
              tunnel: w564 -> [w577 w583]
              tunnel: w565 -> [w575 w582]
              tunnel: [w573 w578] -> w568
              tunnel: [w571 w581] -> w567
              tunnel: w563 -> [w572 w580]
              tunnel: w566 -> [w574 w579]
              frame 1 {
                n302 = Path To String(path=w577) -> (string=w576:string)
                n303 = Open VI Reference(type specifier VI Refnum (for type only)=w572, application reference (local)=w575, vi path=w576, error in (no error)=w574) -> (vi reference=w573:T4, error out=w571:errorcluster)  [unwired: 2 in]
              }
              frame Default {
                n304 = Open VI Reference(type specifier VI Refnum (for type only)=w580, application reference (local)=w582, vi path=w583, error in (no error)=w579) -> (vi reference=w578:T4, error out=w581:errorcluster)  [unwired: 2 in]
              }
            }
          }
        }
        "loaded func infos" <- w537
        n305 = call "Library Open VI Ref Error Clarifier.vi"("VI path"=w535, "called VI error (no error)"=w538) -> ("error out"=w554:errorcluster)  [unwired: 13 in]
        n306 = call "Library Log Error to Window.vi"("error in (no error)"=w554) -> ("dup error"=w553:errorcluster)  [unwired: 13 in, 1 out]
        n307 = Select(t=w561, s=w553, f=w560) -> (s? t:f=w562:T5[])
      }
      frame "init disable" {
        w628 = u8 2 items=["enabled", "disabled", "grayed"] ("disabled state")
        n308 = property on="open" class="Bool"("Disabled"=w628) -> ()  [unwired: 2 in, 2 out]
        n309 = property on="edit" class="Bool"("Disabled"=w628) -> ()  [unwired: 2 in, 2 out]
      }
      frame "init persist" {
        n310 = flat-sequence {
          frame #0 {
            n311 = call "Libary Persist Position and Controls.vi"("action"=enum16{"save", "load"}."load") -> ()  [unwired: 13 in, 2 out]
          }
          frame #1 {
            # "make sure we have path persistence slots"
            n312 = local read "html paths"() -> (w638:path[])
            n313 = property on="source selection" class="Enum (strict)"() -> ("Number of Items"=w639:u32)  [unwired: 2 in, 2 out]
            n314 = To Long Integer(number=w639) -> (32bit integer=w636:i32)
            n315 = for {
              N: w636 -> [_]
              tunnel: w638 -> [w642]
              tunnel: [w640] -> w637 mode=indexing
              i -> [w641]
              n316 = Index Array(array=w642, index=w641) -> (element=w640:path)
            }
            n317 = local write "html paths"(w637) -> ()
          }
        }
        n318 = Build Array (concatenate)(t_LuaVIEW_Function_Manager_States."match sizes" ("states"), w634) -> (w631:T5[])
      }
      frame "init source" {
        w648 = T5[] [enum."refresh source"] items=["empty queue", "update source", "set source", "refresh source", "cleanup registry", "update list", "update ablement", "show", "export", "open", "edit", "fetch loaded", "query base", "query llb", "recurse base", "query library", "parse library", "match sizes", "initialize", "init refs", "init disable", "init persist", "init source", "cleanup", "stop"] ("Array Constant")
        n319 = Reshape Array(w649, 0 ("dimension size")) -> (w647:T8[])
        n320 = Reshape Array(w644, 0 ("dimension size")) -> (w643:i32[])
        n321 = Build Array (concatenate)(w648, w650) -> (w651:T5[])
      }
      frame "cleanup" {
        w660 = T5[] [enum."stop"] items=["empty queue", "update source", "set source", "refresh source", "cleanup registry", "update list", "update ablement", "show", "export", "open", "edit", "fetch loaded", "query base", "query llb", "recurse base", "query library", "parse library", "match sizes", "initialize", "init refs", "init disable", "init persist", "init source", "cleanup", "stop"] ("Array Constant")
        n322 = local read "loaded func infos"() -> (w653:T4)
        n323 = local read "cleanup registry"() -> (w652:T1)
        n324 = local read "get func doc"() -> (w654:T3)
        n325 = property on="function list" class="MCListbox (strict)"("Item Names"=string[][] []) -> ()  [unwired: 2 in, 2 out]
        n326 = call "obj_Library Session.vi"("method"=t_Library_Session_Methods."delist") -> ()  [unwired: 11 in, 4 out]
        n327 = call "Libary Persist Position and Controls.vi"("action"=enum16{"save", "load"}."save") -> ()  [unwired: 13 in, 2 out]
        n328 = Close Reference(reference=w654) -> ()  [unwired: 1 in, 1 out]
        n329 = Close Reference(reference=w653) -> ()  [unwired: 1 in, 1 out]
        n330 = Close Reference(reference=w652) -> ()  [unwired: 1 in, 1 out]
      }
      frame "stop" {
        n331 = invoke class="VI" method="FP.Close"() -> ()  [unwired: 3 in, 3 out]
      }
    }
  }
